vi "Connect.vi"(6 "remote_port":u16, 7 "host_port":u16, 8 "error in (no error)":errorcluster, 9 "remote_address":string, 10 "host_address":string, 11 "Socket.TCP in":refnum<class "Socket.TCP.lvclass">) -> (0 "error out":errorcluster, 3 "Socket.TCP out":refnum<class "Socket.TCP.lvclass">)   [LabVIEW 2014, in "Socket.lvlib" / "Socket.TCP.lvclass"]
doc: "socket.TCP Connect established a remote TCP connecton.\n\nstring host_address is the optional address of the host. Not used by Connect but saved in the class properties to be used later.\n\nu16 host_port is the optional port to connect to on the host. It is recommended to leave this unconnected to allow the OS to choose the best local port to use. Otherwise, the system's TIME-WAIT state makes recently closed ports unavailable for a while. Allowing the OS to choose the port number allows for quick re-connect.\n\nstring remote_address the address to connect to on the remote target.\n\nstring remote_port is the port to connect to on the remote target."
uses:
  Socket.TCP.lvclass
  Socket.Base/Socket.Base.lvclass/Socket.Base.ctl
  Socket.TCP.lvclass/Socket.TCP.ctl
  Accessors/Write host_address.vi
  Accessors/Write host_port.vi
  Accessors/Write remote_address .vi
  Accessors/Write remote_port .vi
  Accessors/Write tcp _refnum.vi
  Socket.Base/Accessors/Write connected.vi
  Socket.Base/Accessors/Read connected.vi
  Socket.Base/Accessors/Read timeout.vi
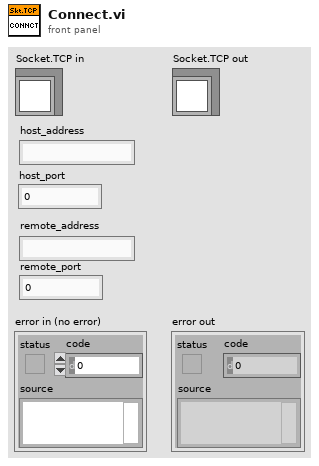
[diagram p1: front panel]
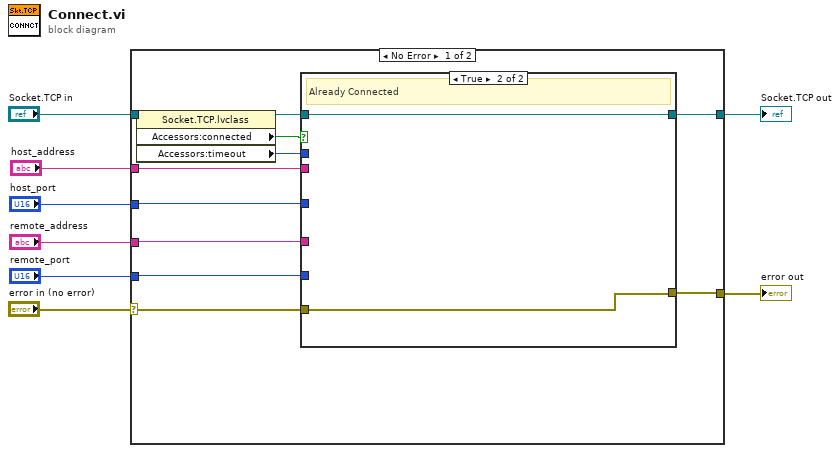
[diagram p0: block diagram]
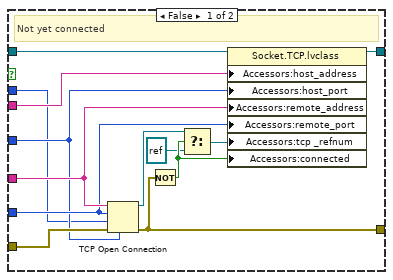
[diagram p2: hidden frame]
diagram:
  n1 = case shown="No Error" "error in (no error)" {
    selector: "error in (no error)" -> [w18 w36]
    tunnel: [w11 w36] -> w7
    tunnel: [w17 w35] -> w5
    tunnel: "Socket.TCP in" -> [w19 w35]
    tunnel: "host_address" -> [w16 _]
    tunnel: "remote_address" -> [w15 _]
    tunnel: "remote_port" -> [w14 _]
    tunnel: "host_port" -> [w13 _]
    frame No Error {
      n2 = property class="Socket.TCP.lvclass"(reference=w19) -> (reference out=w12:refnum<class "Socket.TCP.lvclass">, "Accessors:connected"=w9:bool, "Accessors:timeout"=w10:i32)  [unwired: 1 in, 1 out]
      n3 = case shown="True" w9 {
        tunnel: w18 -> [w32 w33]
        tunnel: [w31 w34] -> w17
        tunnel: w16 -> [w30 _]
        tunnel: w15 -> [w29 _]
        tunnel: w14 -> [w28 _]
        tunnel: w13 -> [w27 _]
        tunnel: w12 -> [w26 w34]
        tunnel: [w25 w33] -> w11
        tunnel: w10 -> [w20 _]
        frame False {
          # "Not yet connected"
          n4 = TCP Open Connection(address=w29, remote port or service name=w28, timeout ms (60000)=w20, local port=w27, error in (no error)=w32) -> (connection ID=w22:refnum<k5>, error out=w25:errorcluster)
          n5 = Not(x=w25) -> (.not. x?=w23:bool)
          n6 = Select(t=w22, s=w23, f=refnum<k5> refnum) -> (s? t:f=w24:refnum<k5>)
          n7 = property class="Socket.TCP.lvclass"(reference=w26, "Accessors:host_address"=w30, "Accessors:host_port"=w27, "Accessors:remote_address "=w29, "Accessors:remote_port "=w28, "Accessors:tcp _refnum"=w24, "Accessors:connected"=w23) -> (reference out=w31:refnum<class "Socket.TCP.lvclass">)  [unwired: 1 in, 1 out]
        }
        frame True {
          # "Already Connected"
        }
      }
    }
    frame Error {
    }
  }
  "error out" <- w7
  "Socket.TCP out" <- w5
